vi "PageEngine.vi"   [LabVIEW 2016, in "PanelSplitForDisplay.lvclass"]
uses:
  PanelSplitForDisplay.lvclass
  <vilib>/Utility/error.llb/DialogType.ctl
  Architecture/Queue Management/ARC_Queue Create_Single.vi
  Architecture/Queue Management/ARC_Queue Remove Element.vi
  Architecture/Queue Management/ARC_Queue Insert Element.vi
  Architecture/Queue Management/ARC_Queue Destroy_Single.vi
  PanelRootNode/PanelRootNode.lvclass
types:
  T1 = cluster{"error":errorcluster, "Event":string, "Data":variant, "Q_Local":string, "PageNames":string[], "PageVIRefs":refnum<vi>[], "PageTreeTags":string[], "CurrentPage":string, "PageVIPath":path, "PanelUIQName":string, "Send":cluster{"VI*ToSend":refnum<vi>, "EventToSend":string, "DataToSend":variant}, "PageCtr*":refnum<vi>, "SubPanel*":refnum<vi>}
  T2 = cluster{"Page":refnum<vi>, "SubPanel":refnum<vi>}
  T3 = typedef "DialogType.ctl" = u16
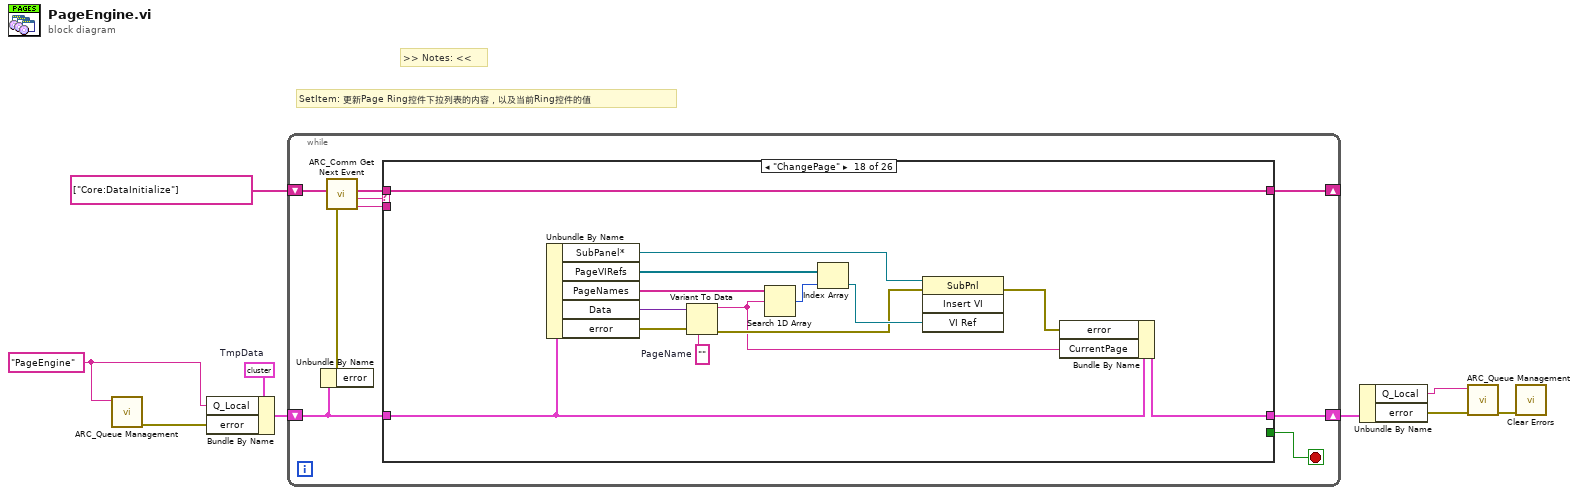
[diagram p0: block diagram]
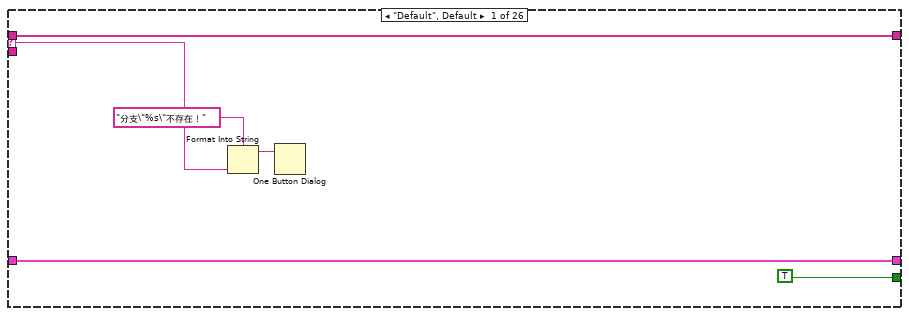
[diagram p2: hidden frame]
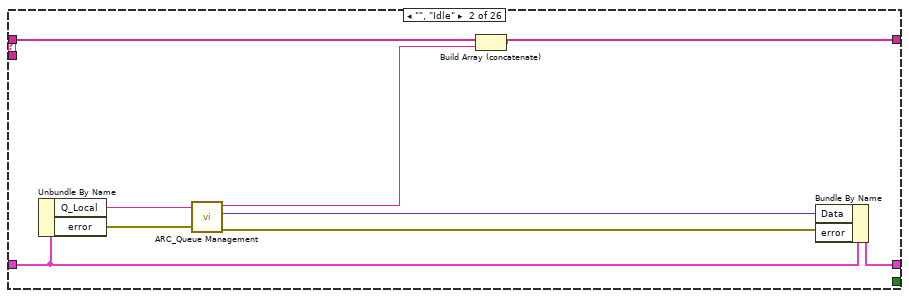
[diagram p3: hidden frame]
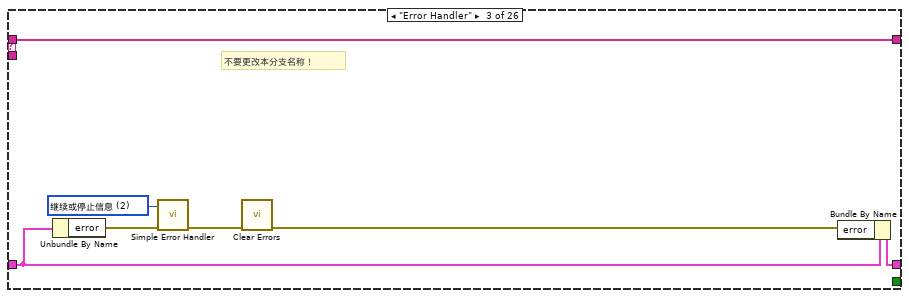
[diagram p4: hidden frame]
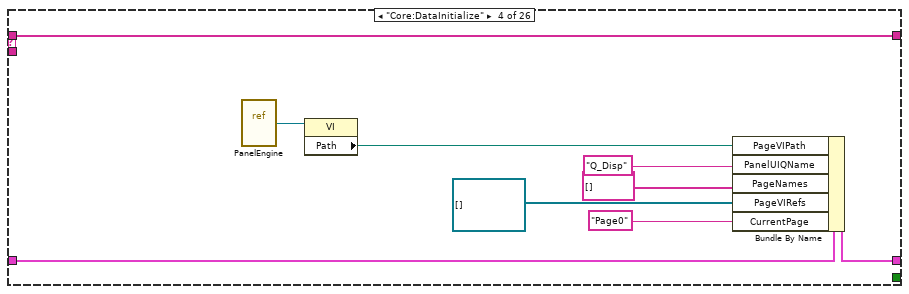
[diagram p5: hidden frame]
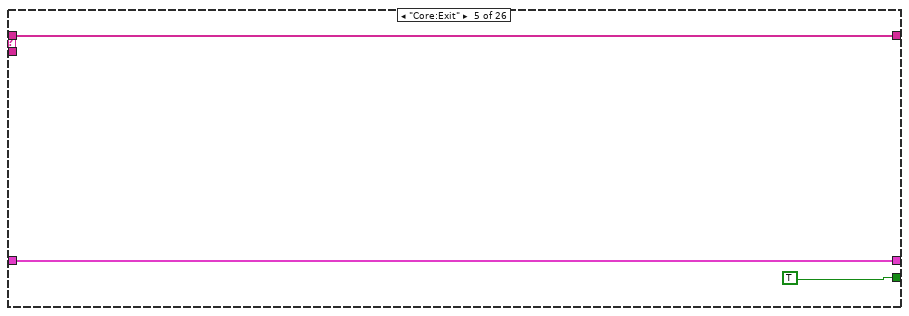
[diagram p6: hidden frame]
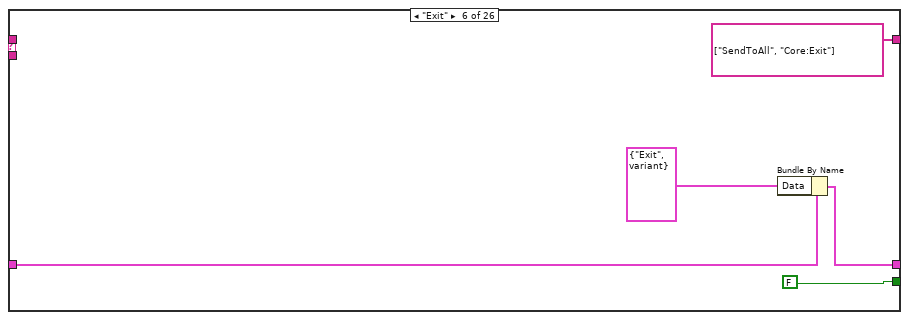
[diagram p7: hidden frame]
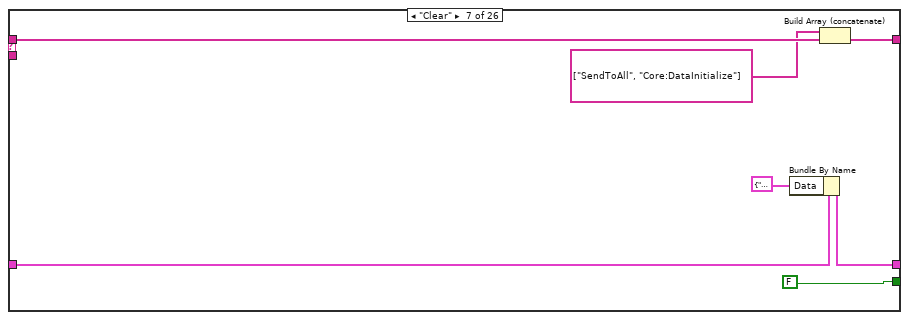
[diagram p8: hidden frame]
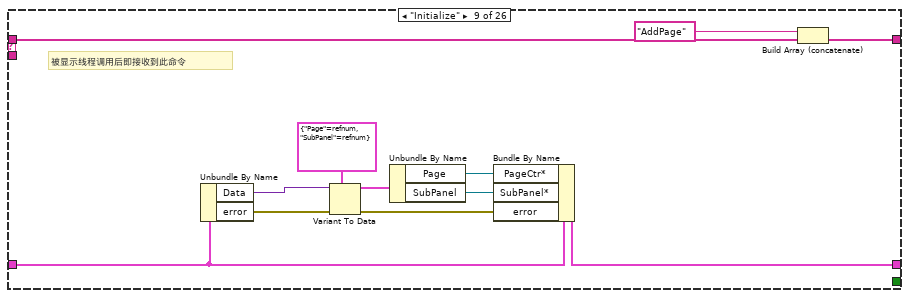
[diagram p10: hidden frame]
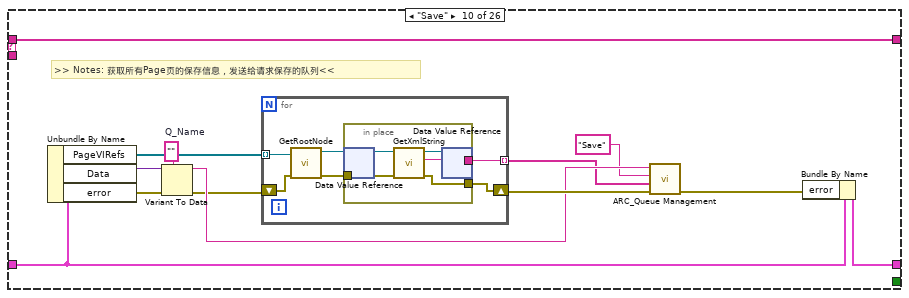
[diagram p11: hidden frame]
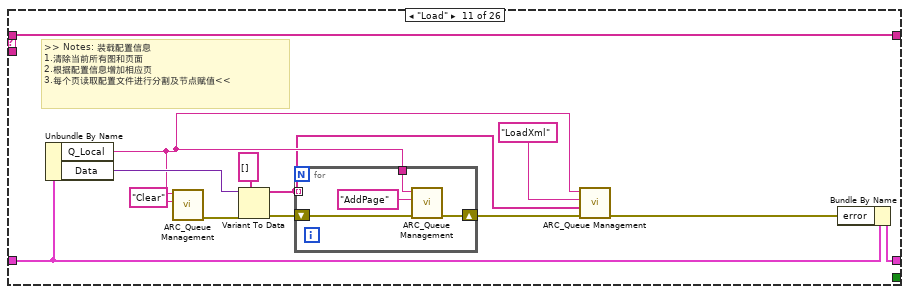
[diagram p12: hidden frame]
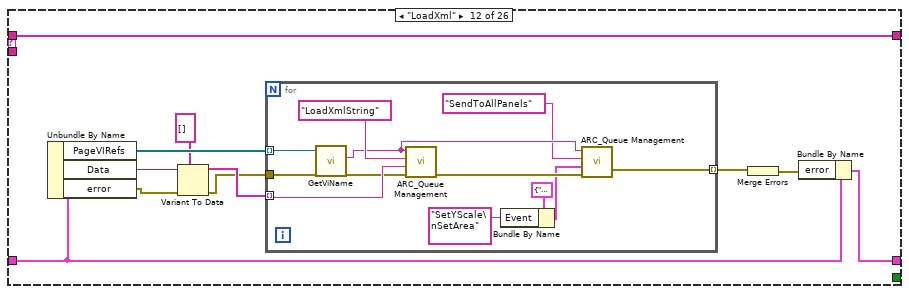
[diagram p13: hidden frame]
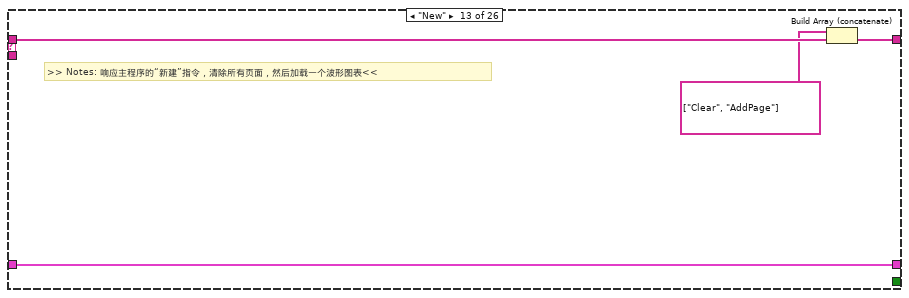
[diagram p14: hidden frame]
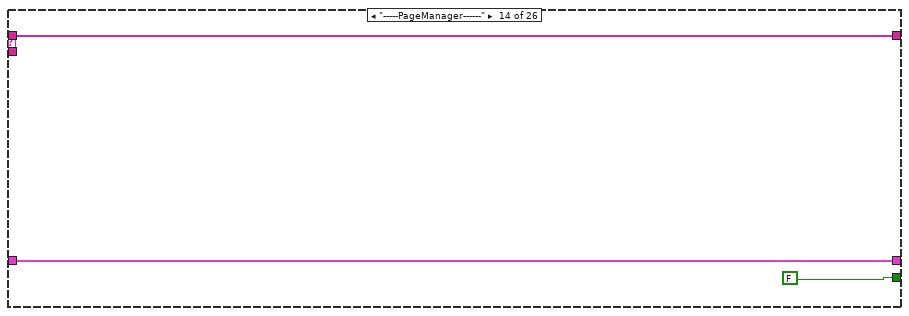
[diagram p15: hidden frame]
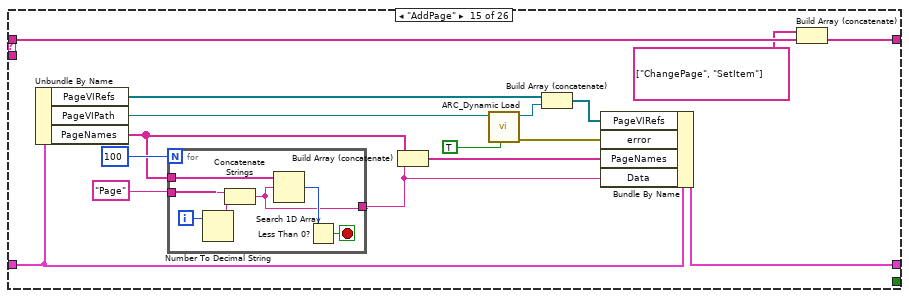
[diagram p16: hidden frame]
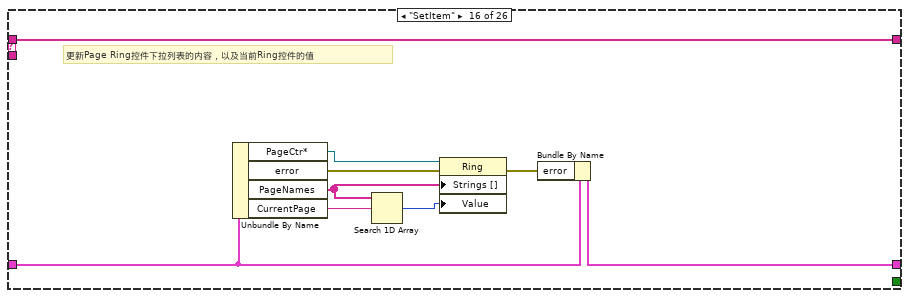
[diagram p17: hidden frame]
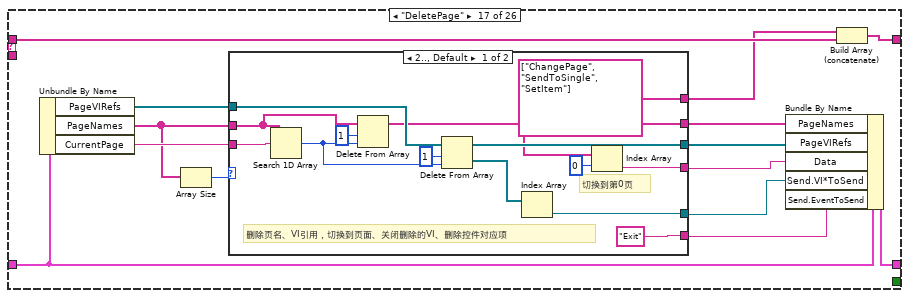
[diagram p18: hidden frame]
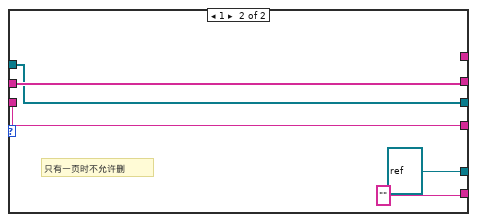
[diagram p19: hidden frame]
diagram:
  w7 = T1 {"error"={"status"=FALSE, "code"=0, "source"=""}, "Event"="", "Data"=variant, "Q_Local"="", "PageNames"=[], "PageVIRefs"=[], "PageTreeTags"=[], "CurrentPage"="", "PageVIPath"=path "", "PanelUIQName"="", "Send"={"VI*ToSend"=refnum, "EventToSend"="", "DataToSend"=variant}, "PageCtr*"=refnum, "SubPanel*"=refnum}  # TmpData
  w5 = "PageEngine" ("QueueName")
  # "SetItem: 更新Page Ring控件下拉列表的内容，以及当前Ring控件的值"
  # ">> Notes: <<"
  n1 = call-poly "ARC_Queue Management.vi"("Queue Name"=w5) -> ("error out"=w3:errorcluster)  [unwired: 8 in, 2 out]
  n2 = Bundle By Name(cluster=w7, "Q_Local"=w5, "error"=w3) -> (w6:T1)
  n3 = while {
    shift-right: [w14] -> w8
    shift-left: w6 -> [w15]
    shift-right: [w13] -> _
    shift-left: string[] ["Core:DataInitialize"] ("event queue in") -> [w12]
    stop <- w17 stop-if-true
    n4 = Unbundle By Name(w15) -> ("error"=w16:errorcluster)
    n5 = call "ARC_Comm Get Next Event.vi"("error in (no error)"=w16, "event queue in"=w12) -> ("prev event"=w18:string, "next event"=w10:string, "event queue out"=w11:string[])  [unwired: 4 in]
    n6 = case shown="\"ChangePage\"" w10 {
      selector: w10 -> [w22 _ _ _ _ _ _ _ _ _ _ _ _ _ _ _ _ _ _ _ _ _ _ _ _ _]
      tunnel: w11 -> [w23 w27 w40 w49 w50 _ w60 w66 w69 w91 w103 w120 w144 w146 w151 w172 w183 w227 w229 w240 w251 w254 w276 w278 w290 w299]
      tunnel: w18 -> [_ _ _ _ _ _ _ _ _ _ _ _ _ _ _ _ _ _ _ _ _ _ _ _ _ _]
      tunnel: [TRUE _ _ _ TRUE FALSE FALSE _ _ _ _ _ _ FALSE _ _ _ _ _ _ _ _ _ _ _ _] -> w17
      tunnel: w15 -> [w24 w30 w36 w48 w51 w55 w62 w65 w76 w89 w107 w129 w145 w147 w162 w176 w192 w217 w228 w231 w242 w260 w271 w277 w281 w302]
      tunnel: [w24 w32 w35 w47 w51 w54 w61 w65 w75 w88 w105 w128 w145 w147 w160 w175 w189 w216 w228 w230 w241 w256 w269 w277 w280 w300] -> w14
      tunnel: [w23 w25 w40 w49 w50 string[] ["SendToAll", "Core:Exit"] ("event queue out") w59 w66 w68 w91 w103 w120 w143 w146 w150 w172 w182 w227 w229 w240 w251 w253 w276 w278 w290 w298] -> w13
      frame "Default", Default {
        n7 = Format Into String(format string="分支\"%s\"不存在！" ("格式字符串"), w22) -> (resulting string=w21:string)  [unwired: 2 in, 1 out]
        n8 = One Button Dialog(message=w21) -> ()  [unwired: 1 in, 1 out]
      }
      frame "", "Idle" {
        n9 = Unbundle By Name(w30) -> ("Q_Local"=w29:string, "error"=w28:errorcluster)
        n10 = call-poly "ARC_Queue Management.vi"("error in (no error)"=w28, "Queue Name(unamed)"=w29) -> ("error out"=w33:errorcluster, "Data"=w31:variant, "Event"=w26:string)  [unwired: 6 in, 1 out]
        n11 = Build Array (concatenate)(w27, w26) -> (w25:string[])
        n12 = Bundle By Name(cluster=w30, "Data"=w31, "error"=w33) -> (w32:T1)
      }
      frame "Error Handler" {
        w34 = T3 2 items=["无对话框", "确定信息", "继续或停止信息", "确定信息＋警告", "继续/停止+警告"] ("type of dialog (OK msg:1)")
        # "不要更改本分支名称！"
        n13 = Unbundle By Name(w36) -> ("error"=w37:errorcluster)
        n14 = call <vilib>:"Simple Error Handler.vi"("type of dialog (OK msg:1)"=w34, "error in (no error)"=w37) -> ("error out"=w38:errorcluster)  [unwired: 3 in, 4 out]
        n15 = call <vilib>:"Clear Errors.vi"("error in (no error)"=w38) -> ("error out"=w39:errorcluster)  [unwired: 5 in, 1 out]
        n16 = Bundle By Name(cluster=w36, "error"=w39) -> (w35:T1)
      }
      frame "Core:DataInitialize" {
        n17 = vi-ref "PanelEngine.vi"() -> (w45:refnum<vi>)
        n18 = property class="VI"(reference=w45) -> ("Path"=w44:path)  [unwired: 1 in, 2 out]
        n19 = Bundle By Name(cluster=w48, "PageVIPath"=w44, "PanelUIQName"="Q_Disp", "PageNames"=string[] [], "PageVIRefs"=refnum<vi>[] [], "CurrentPage"="Page0") -> (w47:T1)
      }
      frame "Core:Exit" {
      }
      frame "Exit" {
        n20 = Bundle By Name(cluster=w55, "Data"=cluster{string, "变体":variant} {"Exit", "变体"=variant}) -> (w54:T1)
      }
      frame "Clear" {
        n21 = Bundle By Name(cluster=w62, "Data"=cluster{string, "变体":variant} {"Exit", "变体"=variant}) -> (w61:T1)
        n22 = Build Array (concatenate)(string[] ["SendToAll", "Core:DataInitialize"] ("event queue in"), w60) -> (w59:string[])
      }
      frame "--------Init------------" {
      }
      frame "Initialize" {
        # "被显示线程调用后即接收到此命令"
        n23 = Unbundle By Name(w76) -> ("Data"=w78:variant, "error"=w70:errorcluster)
        n24 = Variant To Data(error in=w70, type=T2 {"Page"=refnum, "SubPanel"=refnum}, Variant=w78) -> (data=w74:T2, error out=w71:errorcluster)
        n25 = Unbundle By Name(w74) -> ("Page"=w73:refnum<vi>, "SubPanel"=w72:refnum<vi>)
        n26 = Bundle By Name(cluster=w76, "PageCtr*"=w73, "SubPanel*"=w72, "error"=w71) -> (w75:T1)
        n27 = Build Array (concatenate)("AddPage" ("State(s) in Front (\"\")"), w69) -> (w68:string[])
      }
      frame "Save" {
        w86 = ""  # Q_Name
        # ">> Notes: 获取所有Page页的保存信息，发送给请求保存的队列<<"
        n28 = Unbundle By Name(w89) -> ("PageVIRefs"=w90:refnum<vi>[], "Data"=w87:variant, "error"=w79:errorcluster)
        n29 = Variant To Data(error in=w79, type=w86, Variant=w87) -> (data=w83:string, error out=w80:errorcluster)
        n30 = for {
          tunnel: w90 -> [w97] mode=indexing
          tunnel: [w94] -> w82 mode=indexing
          shift-right: [w93] -> w85
          shift-left: w80 -> [w92]
          n31 = call "GetRootNode.vi"("error in"=w92, "vi*"=w97) -> ("error out"=w95:errorcluster, "RootNode*"=w96:refnum<data-value>)  [unwired: 8 in]
          n32 = in-place {
            in-place-border: w95 -> [w100]
            in-place-border: [w99] -> w93
            in-place-border: [w98] -> w94
            n33 = in-place-dvr #1(w96) -> (w102:refnum<class "PanelRootNode.lvclass">)  [unwired: 1 out]
            n34 = call-dynamic "GetXmlString.vi"("error in"=w100, "PanelRootNode 输入"=w102) -> ("error out"=w99:errorcluster, "XML"=w98:string, "PanelRootNode 输出"=w101:refnum<class "PanelRootNode.lvclass">)  [unwired: 7 in]
            n35 = in-place-dvr #1(w101) -> ()  [unwired: 2 out]
          }
        }
        n36 = call-poly "ARC_Queue Management.vi"("error in (no error)"=w85, "Data"=w82, "Event"="Save", "Queue Name(unamed)"=w83) -> ("error out"=w84:errorcluster)  [unwired: 6 in, 1 out]
        n37 = Bundle By Name(cluster=w89, "error"=w84) -> (w88:T1)
      }
      frame "Load" {
        # ">> Notes: 装载配置信息\n1.清除当前所有图和页面\n2.根据配置信息增加相应页\n3.每个页读取配置文件进行分割及节点赋值<<"
        n38 = Unbundle By Name(w107) -> ("Q_Local"=w109:string, "Data"=w114:variant)
        n39 = call-poly "ARC_Queue Management.vi"("Event"="Clear", "Queue Name(unamed)"=w109) -> ("error out"=w112:errorcluster)  [unwired: 8 in, 1 out]
        n40 = Variant To Data(error in=w112, type=string[] [], Variant=w114) -> (data=w104:string[], error out=w111:errorcluster)
        n41 = for {
          tunnel: w109 -> [w118]
          tunnel: w104 -> [_] mode=indexing
          shift-right: [w116] -> w110
          shift-left: w111 -> [w119]
          n42 = call-poly "ARC_Queue Management.vi"("error in (no error)"=w119, "Event"="AddPage", "Queue Name(unamed)"=w118) -> ("error out"=w116:errorcluster)  [unwired: 7 in, 1 out]
        }
        n43 = call-poly "ARC_Queue Management.vi"("error in (no error)"=w110, "Data"=w104, "Event"="LoadXml", "Queue Name(unamed)"=w109) -> ("error out"=w106:errorcluster)  [unwired: 6 in, 1 out]
        n44 = Bundle By Name(cluster=w107, "error"=w106) -> (w105:T1)
      }
      frame "LoadXml" {
        n45 = Unbundle By Name(w129) -> ("PageVIRefs"=w130:refnum<vi>[], "Data"=w125:variant, "error"=w121:errorcluster)
        n46 = Variant To Data(error in=w121, type=string[] [], Variant=w125) -> (data=w124:string[], error out=w122:errorcluster)
        n47 = for {
          tunnel: w130 -> [w141] mode=indexing
          tunnel: w124 -> [w140] mode=indexing
          tunnel: [w137] -> w127 mode=indexing
          tunnel: w122 -> [w131]
          n48 = call "GetViName.vi"("VI*"=w141) -> ("VI Name"=w136:string)  [unwired: 9 in, 1 out]
          n49 = call-poly "ARC_Queue Management.vi"("error in (no error)"=w131, "Data"=w140, "Event"="LoadXmlString", "Queue Name(unamed)"=w136) -> ("error out"=w138:errorcluster)  [unwired: 6 in, 1 out]
          n50 = Bundle By Name(cluster=cluster{"Event":string, "Data":variant} {"Event"="", "Data"=variant} ("Send"), "Event"="SetYScale\nSetArea") -> (w133:cluster{"Event":string, "Data":variant})
          n51 = call-poly "ARC_Queue Management.vi"("error in (no error)"=w138, "Data"=w133, "Event"="SendToAllPanels", "Queue Name(unamed)"=w136) -> ("error out"=w137:errorcluster)  [unwired: 6 in, 1 out]
        }
        n52 = Merge Errors(w127) -> (w126:errorcluster)
        n53 = Bundle By Name(cluster=w129, "error"=w126) -> (w128:T1)
      }
      frame "New" {
        # ">> Notes: 响应主程序的“新建”指令，清除所有页面，然后加载一个波形图表<<"
        n54 = Build Array (concatenate)(string[] ["Clear", "AddPage"] ("element"), w144) -> (w143:string[])
      }
      frame "-----PageManager------" {
      }
      frame "AddPage" {
        n55 = Unbundle By Name(w162) -> ("PageVIRefs"=w158:refnum<vi>[], "PageVIPath"=w159:path, "PageNames"=w153:string[])
        n56 = for {
          N: 100 -> [_]
          tunnel: w153 -> [w168]
          tunnel: "Page" -> [w171]
          tunnel: [w165] -> w154
          i -> [w170]
          stop <- w166 stop-if-true
          n57 = Number To Decimal String(number=w170) -> (decimal integer string=w169:string)  [unwired: 1 in]
          n58 = Concatenate Strings(w171, w169) -> (w165:string)
          n59 = Search 1D Array(1D array=w168, element=w165) -> (index of element=w167:i32)  [unwired: 1 in]
          n60 = Less Than 0?(x=w167) -> (x < 0?=w166:bool)
        }
        n61 = Build Array (concatenate)(w153, w154) -> (w161:string[])
        n62 = call "ARC_Dynamic Load.vi"("Auto Dispose Ref"=TRUE ("自动销毁引用"), "Vi Path"=w159) -> ("错误输出"=w156:errorcluster, "vi reference"=w157:refnum<vi>)  [unwired: 8 in]
        n63 = Build Array (concatenate)(w158, w157) -> (w155:refnum<vi>[])
        n64 = Bundle By Name(cluster=w162, "PageVIRefs"=w155, "error"=w156, "PageNames"=w161, "Data"=w154) -> (w160:T1)
        n65 = Build Array (concatenate)(string[] ["ChangePage", "SetItem"] ("array"), w151) -> (w150:string[])
      }
      frame "SetItem" {
        # "更新Page Ring控件下拉列表的内容，以及当前Ring控件的值"
        n66 = Unbundle By Name(w176) -> ("PageCtr*"=w180:refnum<vi>, "error"=w174:errorcluster, "PageNames"=w173:string[], "CurrentPage"=w179:string)
        n67 = Search 1D Array(1D array=w173, element=w179) -> (index of element=w178:i32)  [unwired: 1 in]
        n68 = property class="Ring"(reference=w180, error in=w174, "Strings []"=w173, "Value"=w178) -> (error out=w177:errorcluster)  [unwired: 1 out]
        n69 = Bundle By Name(cluster=w176, "error"=w177) -> (w175:T1)
      }
      frame "DeletePage" {
        n70 = Unbundle By Name(w192) -> ("PageVIRefs"=w193:refnum<vi>[], "PageNames"=w188:string[], "CurrentPage"=w194:string)
        n71 = Array Size(array=w188) -> (size(s)=w187:i32)
        n72 = case shown="2.., Default" w187 {
          tunnel: w194 -> [w208 w211]
          tunnel: w193 -> [w206 w212]
          tunnel: [w202 w213] -> w191
          tunnel: [w204 w212] -> w190
          tunnel: w188 -> [w203 w213]
          tunnel: [w201 w211] -> w186
          tunnel: [string[] ["ChangePage", "SendToSingle", "SetItem"] ("element") _] -> w181
          tunnel: [w197 refnum<vi> refnum ("VI引用")] -> w185
          tunnel: ["Exit" ""] -> w184
          frame 2.., Default {
            # "删除页名、VI引用，切换到页面、关闭删除的VI、删除控件对应项"
            # "切换到第0页"
            n73 = Search 1D Array(1D array=w203, element=w208) -> (index of element=w200:i32)  [unwired: 1 in]
            n74 = Delete From Array(array=w203, length=1 ("长度"), index=w200) -> (array with subset deleted=w202:string[])  [unwired: 1 out]
            n75 = Delete From Array(array=w206, length=1 ("长度"), index=w200) -> (deleted portion=w198:refnum<vi>[], array with subset deleted=w204:refnum<vi>[])
            n76 = Index Array(array=w198) -> (element=w197:refnum<vi>)  [unwired: 1 in]
            n77 = Index Array(array=w202, index=0 ("索引")) -> (element=w201:string)
          }
          frame 1 {
            # "只有一页时不允许删"
          }
        }
        n78 = Bundle By Name(cluster=w192, "PageNames"=w191, "PageVIRefs"=w190, "Data"=w186, "Send.VI*ToSend"=w185, "Send.EventToSend"=w184) -> (w189:T1)
        n79 = Build Array (concatenate)(w181, w183) -> (w182:string[])
      }
      frame "ChangePage" {
        w224 = ""  # PageName
        n80 = Unbundle By Name(w217) -> ("SubPanel*"=w214:refnum<vi>, "PageVIRefs"=w222:refnum<vi>[], "PageNames"=w223:string[], "Data"=w226:variant, "error"=w225:errorcluster)
        n81 = Variant To Data(error in=w225, type=w224, Variant=w226) -> (data=w215:string, error out=w219:errorcluster)
        n82 = Search 1D Array(1D array=w223, element=w215) -> (index of element=w221:i32)  [unwired: 1 in]
        n83 = Index Array(array=w222, index=w221) -> (element=w220:refnum<vi>)
        n84 = invoke class="SubPnl" method="Insert VI"(reference=w214, error in=w219, "VI Ref"=w220) -> (error out=w218:errorcluster)  [unwired: 1 in, 3 out]
        n85 = Bundle By Name(cluster=w217, "error"=w218, "CurrentPage"=w215) -> (w216:T1)
      }
      frame "-----PanelManager------" {
      }
      frame "AddPanel" {
        n86 = Unbundle By Name(w231) -> ("PageVIRefs"=w237:refnum<vi>[], "PageNames"=w238:string[], "CurrentPage"=w239:string)
        n87 = Search 1D Array(1D array=w238, element=w239) -> (index of element=w236:i32)  [unwired: 1 in]
        n88 = Index Array(array=w237, index=w236) -> (element=w235:refnum<vi>)
        n89 = call "GetViName.vi"("VI*"=w235) -> ("VI Name"=w234:string)  [unwired: 9 in, 1 out]
        n90 = call-poly "ARC_Queue Management.vi"("Event"="AddPanel", "Queue Name(unamed)"=w234) -> ("error out"=w232:errorcluster)  [unwired: 8 in, 1 out]
        n91 = Bundle By Name(cluster=w231, "error"=w232) -> (w230:T1)
      }
      frame "DeletePanel" {
        n92 = Unbundle By Name(w242) -> ("PageVIRefs"=w248:refnum<vi>[], "PageNames"=w249:string[], "CurrentPage"=w250:string)
        n93 = Search 1D Array(1D array=w249, element=w250) -> (index of element=w247:i32)  [unwired: 1 in]
        n94 = Index Array(array=w248, index=w247) -> (element=w246:refnum<vi>)
        n95 = call "GetViName.vi"("VI*"=w246) -> ("VI Name"=w245:string)  [unwired: 9 in, 1 out]
        n96 = call-poly "ARC_Queue Management.vi"("Event"="DeletePanel", "Queue Name(unamed)"=w245) -> ("error out"=w243:errorcluster)  [unwired: 8 in, 1 out]
        n97 = Bundle By Name(cluster=w242, "error"=w243) -> (w241:T1)
      }
      frame "TransferToSingle" {
        # "转发给当前PAGE的Panel引擎"
        n98 = Unbundle By Name(w260) -> ("PageVIRefs"=w262:refnum<vi>[], "PageNames"=w263:string[], "CurrentPage"=w264:string)
        n99 = Unbundle By Name(w260) -> ("Data"=w267:variant)
        n100 = Variant To Data(type=cluster{"Event":string, "Data":variant} {"Event"="", "Data"=variant}, Variant=w267) -> (data=w265:cluster{"Event":string, "Data":variant}, error out=w255:errorcluster)  [unwired: 1 in]
        n101 = Search 1D Array(1D array=w263, element=w264) -> (index of element=w261:i32)  [unwired: 1 in]
        n102 = Unbundle By Name(w265) -> ("Event"=w258:string, "Data"=w259:variant)
        n103 = Index Array(array=w262, index=w261) -> (element=w257:refnum<vi>)
        n104 = Bundle By Name(cluster=w260, "Send.VI*ToSend"=w257, "Send.EventToSend"=w258, "Send.DataToSend"=w259, "error"=w255) -> (w256:T1)
        n105 = Build Array (concatenate)("SendToSingle" ("State(s) in Front (\"\")"), w254) -> (w253:string[])
      }
      frame "SendToSingle" {
        n106 = Unbundle By Name(w271) -> ("Send.EventToSend"=w272:string, "Send.DataToSend"=w273:variant, "Send.VI*ToSend"=w274:refnum<vi>, "error"=w268:errorcluster)
        n107 = call "GetViName.vi"("VI*"=w274) -> ("VI Name"=w275:string)  [unwired: 9 in, 1 out]
        n108 = call-poly "ARC_Queue Management.vi"("error in (no error)"=w268, "Data"=w273, "Event"=w272, "Queue Name(unamed)"=w275) -> ("error out"=w270:errorcluster)  [unwired: 6 in, 1 out]
        n109 = Bundle By Name(cluster=w271, "error"=w270) -> (w269:T1)
      }
      frame "--------Send----------" {
      }
      frame "SendToAll" {
        # ">> Notes: 发送给所有PanelEngine，不是发送给所有页子节点面板<<"
        n110 = Unbundle By Name(w281) -> ("PageVIRefs"=w289:refnum<vi>[], "Data"=w288:variant, "error"=w283:errorcluster)
        n111 = Variant To Data(error in=w283, type=cluster{string, "Data":variant} {"", "Data"=variant}, Variant=w288) -> (data=w286:cluster{string, "Data":variant}, error out=w282:errorcluster)
        n112 = Unbundle(w286) -> (w285:string, "Data"=w284:variant)
        n113 = for {
          tunnel: w289 -> [w296] mode=indexing
          tunnel: w285 -> [w294]
          tunnel: w284 -> [w293]
          shift-right: [w292] -> w279
          shift-left: w282 -> [w291]
          n114 = call "GetViName.vi"("VI*"=w296) -> ("VI Name"=w295:string)  [unwired: 9 in, 1 out]
          n115 = call-poly "ARC_Queue Management.vi"("error in (no error)"=w291, "Data"=w293, "Event"=w294, "Queue Name(unamed)"=w295) -> ("error out"=w292:errorcluster)  [unwired: 6 in, 1 out]
        }
        n116 = Bundle By Name(cluster=w281, "error"=w279) -> (w280:T1)
      }
      frame "SendToAllPanels" {
        (unwired) cluster{"Event":string, "Data":variant} {"Event"="", "Data"=variant} ("Send")
        # ">> Notes: 发送至所有Page页的所有面板，变体Data的数据结构为包含字符串和变体的簇<<"
        n117 = Unbundle By Name(w302) -> ("Data"=w304:variant)
        n118 = disable-structure shown="\"调用形式如下\"" {
          frame condition #0 {
            n119 = call-poly "ARC_Queue Management.vi"("Data"=cluster{"Event":string, "Data":variant} {"Event"="", "Data"=variant} ("Send"), "Event"="SendToAllPanels", "Queue Name(unamed)"="PageEngine" ("QueueName")) -> ()  [unwired: 7 in, 2 out]
          }
          frame condition #1 (active) {
          }
        }
        n120 = Bundle("SendToAllPanels", "Data"=w304) -> (w301:cluster{string, "Data":variant})  [unwired: 1 in]
        n121 = Build Array (concatenate)("SendToAll" ("State(s) in Front (\"\")"), w299) -> (w298:string[])
        n122 = Bundle By Name(cluster=w302, "Data"=w301) -> (w300:T1)
      }
    }
  }
  n123 = Unbundle By Name(w8) -> ("Q_Local"=w4:string, "error"=w9:errorcluster)
  n124 = call-poly "ARC_Queue Management.vi"("error in (no error)"=w9, "Queue Name(unamed)"=w4) -> ("error out"=w1:errorcluster)  [unwired: 7 in, 2 out]
  n125 = call <vilib>:"Clear Errors.vi"("error in (no error)"=w1) -> ()  [unwired: 5 in, 2 out]
